vi "Immediate Color Wheel.vi"(11 "Setpoint":dbl) -> ()   [LabVIEW 2019]
uses:
  <vilib>/Rock Robotics/WPI/Framework/Command Status Info.ctl
  <vilib>/Rock Robotics/WPI/Framework/Completion Status.ctl
  <vilib>/Rock Robotics/WPI/Framework/Completion Notifier.ctl
  Implementation/Color Wheel Setpoints.ctl
  Implementation/Color Wheel Operations.ctl
panel:
  in  "Description":string
  out "Command Info Out":T1
  in  "Command Info In":T1
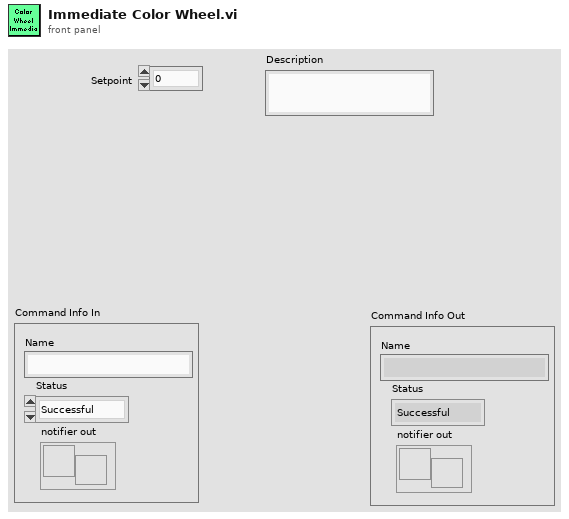
[diagram p1: front panel]
types:
  T1 = typedef "Command Status Info.ctl" = cluster{"Name":string, "Status":T2, "notifier out":T3}
  T2 = typedef "Completion Status.ctl" = enum16{"Successful", "Aborted", "Incomplete"}
  T3 = typedef "Completion Notifier.ctl" = refnum<notifier>
  T4 = typedef "Color Wheel Operations.ctl" = enum16{"Reserve", "Read Current", "Immediate"}
  T5 = typedef "Color Wheel Setpoints.ctl" = cluster{"Operation":T4, "Setpoint":dbl}
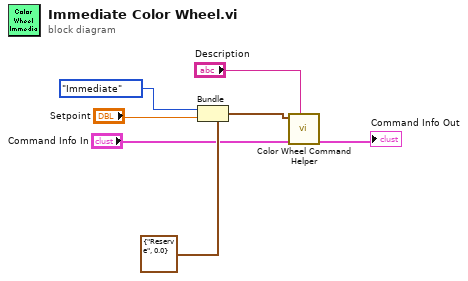
[diagram p0: block diagram]
diagram:
  n1 = Bundle(cluster=T5 {"Operation"=enum."Reserve", "Setpoint"=0.0} ("SubSystem Data"), "Operation"=Color_Wheel_Operations."Immediate", "Setpoint"="Setpoint") -> (w1:T5)
  n2 = call "Color Wheel Command Helper.vi"("Description"="Description", "Command Info In"="Command Info In", "SubSystem Data"=w1) -> ("Command Info Out"=→"Command Info Out":T1)  [unwired: 6 in, 2 out]
